vi "ExampleInstrument.Read Configuration File.vi"(8 "error in (no error)":errorcluster, 11 "Example Instrument in":refnum<class "ExampleInstrument.lvclass">) -> (0 "error out":errorcluster, 3 "Example Instrument out":refnum<class "ExampleInstrument.lvclass">)   [LabVIEW 2016, in "ExampleInstrument.lvclass"]
uses:
  ExampleInstrument.lvclass
  C:/user/patrick/hg/levylab_inst/lvsrc/SMOs/Instrument/Instrument.lvclass
  ExampleInstrument.lvclass/ExampleInstrument.ctl
  lvsrc/SMOs/Instrument/Instrument.lvclass/Instrument.ctl
  lvsrc/SMOs/Configuration/Configuration.lvclass
  lvsrc/SMOs/Instrument/Instrument.lvclass
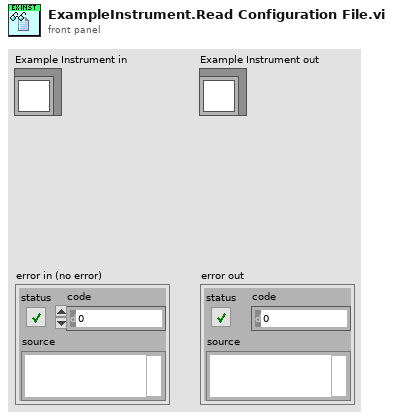
[diagram p1: front panel]
types:
  T1 = typedef "ExampleInstrument.lvclass/ExampleInstrument.Configuration--Cluster.ctl" = cluster{"Example Setting 1":dbl, "Example Setting 2":dbl, "Example Setting 3":string}
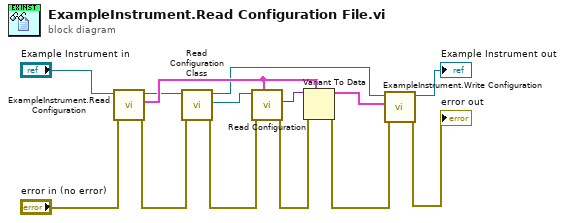
[diagram p0: block diagram]
diagram:
  n1 = call "ExampleInstrument.Read Configuration.vi"("error in (no error)"="error in (no error)", "Example Instrument in"="Example Instrument in") -> ("error out"=w6:errorcluster, "Configuration"=w10:T1, "Example Instrument out"=w8:refnum<class "ExampleInstrument.lvclass">)  [unwired: 7 in]
  n2 = call "Read Configuration Class.vi"("error in (no error)"=w6, "Instrument in"=w8) -> ("error out"=w5:errorcluster, "Configuration.lvclass"=w9:refnum<class "Configuration.lvclass">, "Instrument out"=w7:refnum<class "ExampleInstrument.lvclass">)  [unwired: 7 in]
  n3 = call "Read Configuration.vi"("INI Fomatted Cluster Type"=w10, "error in (no error)"=w5, "Configuration in"=w9) -> ("error out"=w13:errorcluster, "Configuration"=w14:variant)  [unwired: 6 in, 1 out]
  n4 = Variant To Data(error in=w13, type=w10, Variant=w14) -> (data=w12:T1, error out=w11:errorcluster)
  n5 = call "ExampleInstrument.Write Configuration.vi"("error in (no error)"=w11, "Configuration"=w12, "Example Instrument in"=w7) -> ("error out"=→"error out":errorcluster, "Example Instrument out"=→"Example Instrument out":refnum<class "ExampleInstrument.lvclass">)  [unwired: 7 in]
